vi "Draw.vi"(8 "error in (no error)":errorcluster, 10 "2D Picture in":picture, 11 "Rectangle in":refnum<class "Rectangle.lvclass">) -> (0 "error out":errorcluster, 2 "2D Picture out":picture, 3 "Rectangle out":refnum<class "Rectangle.lvclass">)   [LabVIEW 2021, in "Picture2D.lvlib" / "Rectangle.lvclass"]
uses:
  Rectangle.lvclass
  Rectangle.lvclass/Rectangle.ctl
  Color/Color.lvclass
  Polygone/Polygone.lvclass
  Pen/Pen.lvclass
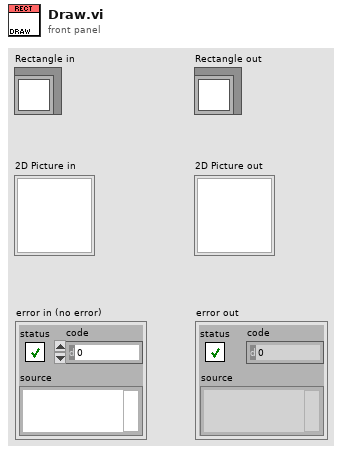
[diagram p1: front panel]
types:
  T1 = cluster{"Width":u16, "Style":enum32{"Solid", "Dash", "Dot", "DashDot", "DashDotDot"}}
  T2 = cluster{"left":i16, "top":i16, "right":i16, "bottom":i16}
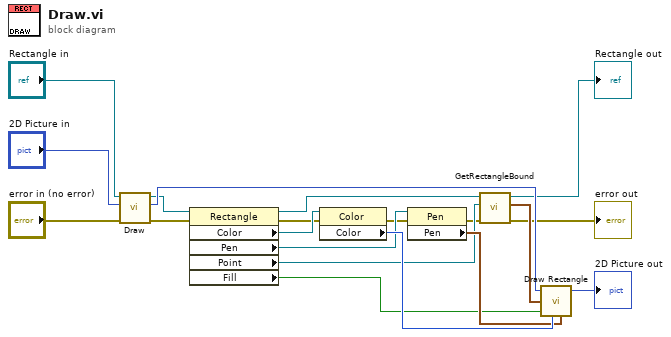
[diagram p0: block diagram]
diagram:
  n1 = call-parent "Draw.vi"("error in (no error)"="error in (no error)", "2D Picture in"="2D Picture in", "Shape in"="Rectangle in") -> ("error out"=w3:errorcluster, "2D Picture out"=w17:picture, "Shape out"=w10:refnum<class "Rectangle.lvclass">)  [unwired: 6 in]
  n2 = property class="Rectangle"(reference=w10, error in=w3) -> (reference out=w8:refnum<class "Rectangle.lvclass">, error out=w5:errorcluster, "Color"=w15:refnum<class "Color.lvclass">, "Pen"=w13:refnum<class "Pen.lvclass">, "Point"=w11:refnum<class "Point.lvclass">, "Fill"=w1:bool)
  n3 = property class="Color"(reference=w15, error in=w5) -> (error out=w4:errorcluster, "Color"=w14:u32)  [unwired: 1 out]
  n4 = property class="Pen"(reference=w13, error in=w4) -> (error out=w2:errorcluster, "Pen"=w12:T1)  [unwired: 1 out]
  n5 = call "GetRectangleBound.vi"("error in (no error)"=w2, "Point"=w11, "Rectangle in"=w8) -> ("error out"=→"error out":errorcluster, "rect"=w9:T2, "Rectangle out"=→"Rectangle out":refnum<class "Rectangle.lvclass">)  [unwired: 6 in]
  n6 = call <vilib>:"Draw Rectangle.vi"("picture"=w17, "rect"=w9, "fill?(F)"=w1, "color(black)"=w14, "pen"=w12) -> ("new picture"=→"2D Picture out":picture)  [unwired: 4 in]
